vi "Day 5 - If You Give A Seed A Fertilizer.vi"() -> ()   [LabVIEW 2020, in "AoC 2023.lvlib"]
uses:
  AoC 2023.lvlib
  <vilib>/Utility/miscctls.llb/LVMapReplaceAction.ctl
panel:
  out "Puzzle Part-2 Answer":string
  out "Puzzle Answer":string
  in  "Puzzle Input":string="seeds: 79 14 55 13\n\nseed-to-soil map:\n50 98 2\n52 50 48\n\nsoil-to-fertilizer map:\n0 15 37\n37 52 2\n39 0 15\n\nfertilizer-to-water map:\n49 53 8\n0 11 42\n42 0 7\n57 7 4\n\nwater-to-light map:\n88 18 7\n18 25 70\n\nlight-to-temperature map:\n45 77 23\n81 45 19\n68 64 13\n\ntemperature-to-humidity map:\n0 69 1\n1 0 69\n\nhumidity-to-location map:\n60 56 37\n56 93 4"
  # "Enter the Puzzle Input and run the VI"
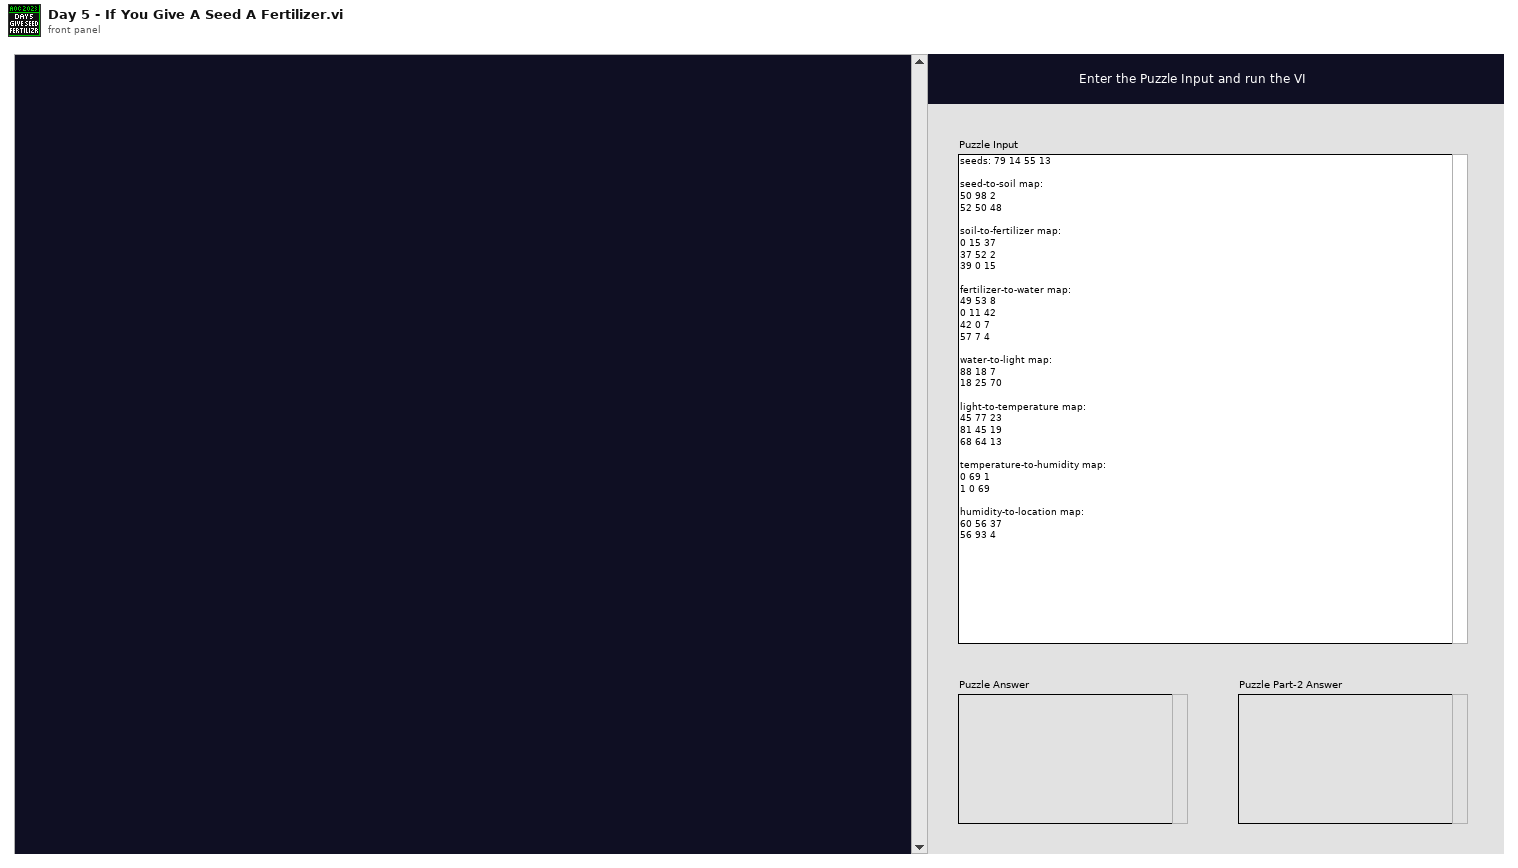
[diagram p1: front panel]
types:
  T1 = map{i32, cluster{"src range start":u64, "src range end":u64, "dst start":u64}[]}
  T2 = typedef "LVMapReplaceAction.ctl" = enum32{"Modify Entry only if found", "Add or Modify Entry", "Delete Entry"}
  T3 = cluster{"src range start":u64, "src range end":u64, "dst start":u64}[]
  T4 = cluster{"src range start":u64, "src range end":u64, "dst start":u64}
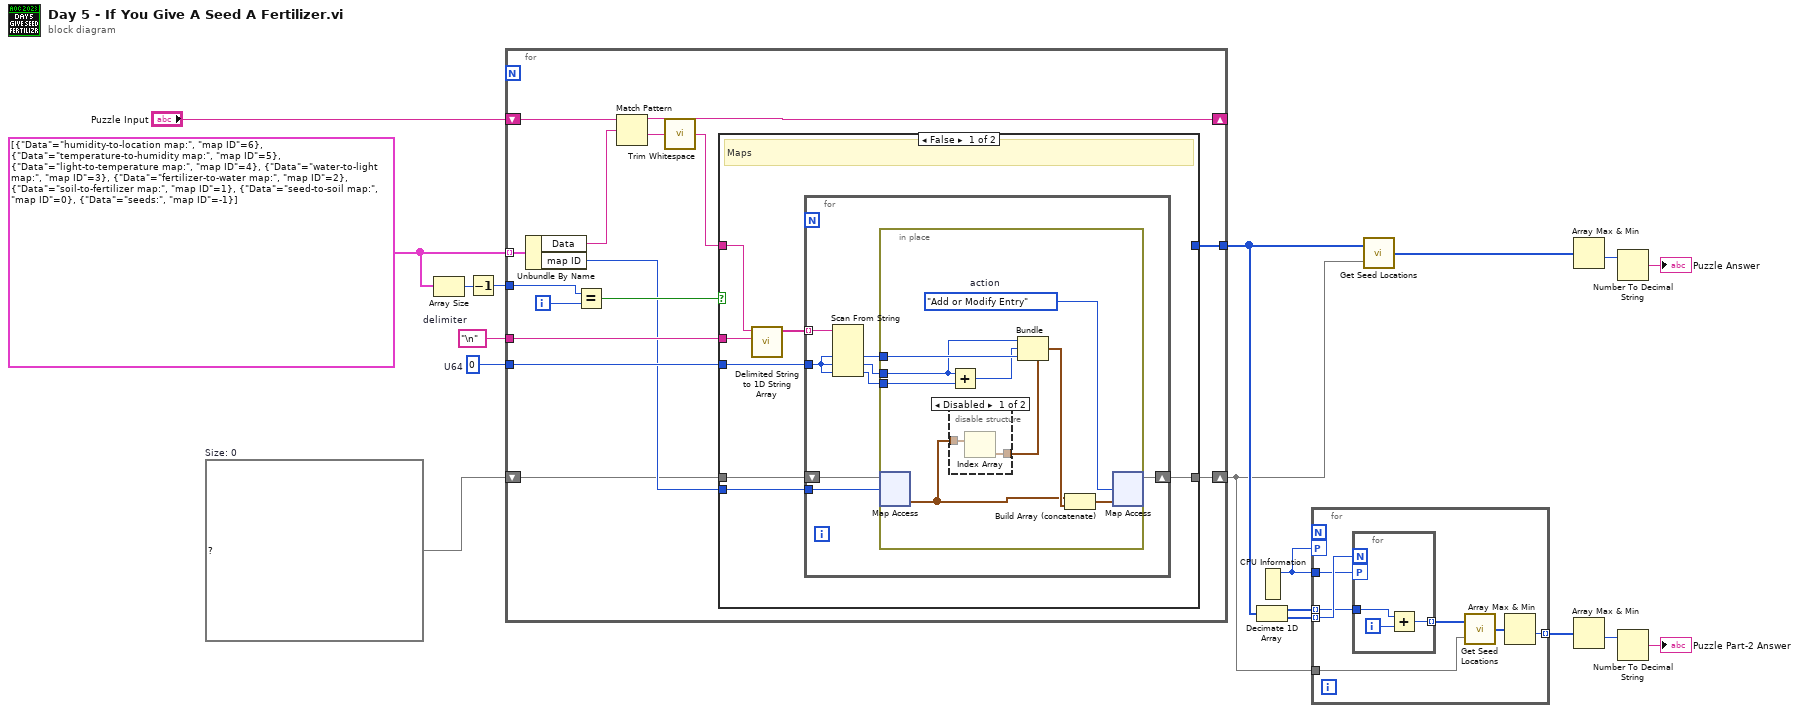
[diagram p0: block diagram]
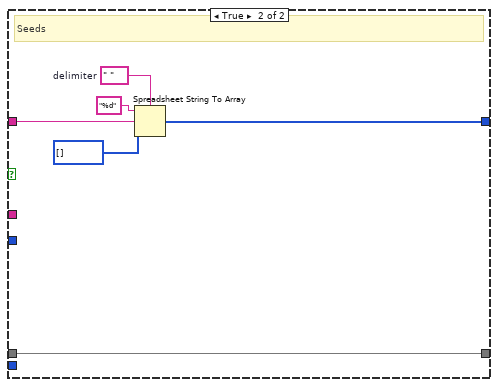
[diagram p3: hidden frame]
diagram:
  w10 = T1 {}  # Size: 0
  w11 = cluster{"Data":string, "map ID":i32}[] [{"Data"="humidity-to-location map:", "map ID"=6}, {"Data"="temperature-to-humidity map:", "map ID"=5}, {"Data"="light-to-temperature map:", "map ID"=4}, {"Data"="water-to-light map:", "map ID"=3}, {"Data"="fertilizer-to-water map:", "map ID"=2}, {"Data"="soil-to-fertilizer map:", "map ID"=1}, {"Data"="seed-to-soil map:", "map ID"=0}, {"Data"="seeds:", "map ID"=-1}]
  w15 = u64 0  # U64
  w16 = "\n"  # delimiter
  n1 = Array Size(array=w11) -> (size(s)=w14:i32)
  n2 = Decrement(x=w14) -> (x-1=w13:i32)
  n3 = for {
    shift-right: [w32] -> _
    shift-left: "Puzzle Input" -> [w33]
    tunnel: w11 -> [w23] mode=indexing
    tunnel: w16 -> [w30]
    tunnel: w15 -> [w28]
    tunnel: w13 -> [w27]
    tunnel: [w24] -> w7
    shift-right: [w20] -> w4
    shift-left: w10 -> [w19]
    i -> [w26]
    n4 = Unbundle By Name(w23) -> ("Data"=w22:string, "map ID"=w21:i32)
    n5 = Equal?(x=w27, y=w26) -> (x = y?=w25:bool)
    n6 = Match Pattern(string=w33, regular expression=w22) -> (before substring=w32:string, after substring=w31:string)  [unwired: 1 in, 2 out]
    n7 = call <vilib>:"Trim Whitespace.vi"("string"=w31) -> ("trimmed string"=w29:string)  [unwired: 1 in]
    n8 = case shown="False" w25 {
      tunnel: w30 -> [w40 _]
      tunnel: w29 -> [w39 w62]
      tunnel: w28 -> [w37 _]
      tunnel: [_ w61] -> w24
      tunnel: w21 -> [w36 _]
      tunnel: [w35 w60] -> w20
      tunnel: w19 -> [w34 w60]
      frame False {
        # "Maps"
        n9 = call <vilib>:"Delimited String to 1D String Array.vi"("delimiter"=w40, "delimited string"=w39) -> ("string array"=w38:string[])  [unwired: 9 in]
        n10 = for {
          tunnel: w38 -> [w48] mode=indexing
          tunnel: w37 -> [w47]
          tunnel: w36 -> [w43]
          shift-right: [w42] -> w35
          shift-left: w34 -> [w41]
          n11 = Scan From String(input string=w48, default 1=w47, default 2=w47, default 3=w47) -> (output 1=w46:u64, output 2=w45:u64, output 3=w44:u64)  [unwired: 3 in, 3 out]
          n12 = in-place {
            in-place-border: w46 -> [w51]
            in-place-border: w45 -> [w50]
            in-place-border: w44 -> [w57]
            w54 = LVMapReplaceAction."Add or Modify Entry"  # action
            n13 = in-place-map #1(w41, w43) -> (w53:T3)  [unwired: 1 in, 1 out]
            n14 = Add(x=w50, y=w57) -> (x+y=w49:u64)
            n15 = disable-structure shown="Disabled" {
              disable-tunnel: w53 -> [w59 _]
              disable-tunnel: [w58 _] -> w52
              frame Disabled {
                n16 = Index Array(array=w59) -> (element=w58:T4)  [unwired: 1 in]
              }
              frame Enabled {
              }
            }
            n17 = Bundle(cluster=w52, "src range start"=w50, "src range end"=w49, "dst start"=w51) -> (w56:T4)
            n18 = Build Array (concatenate)(w53, w56) -> (w55:T3)
            n19 = in-place-map #1(w55, w54) -> (w42:T1)  [unwired: 2 out]
          }
        }
      }
      frame True {
        w65 = " "  # delimiter
        # "Seeds"
        n20 = Spreadsheet String To Array(delimiter (Tab)=w65, format string="%d", spreadsheet string=w62, array type (2D Dbl)=u64[] []) -> (array=w61:u64[])
      }
    }
  }
  n21 = Decimate 1D Array(w7) -> (w6:u64[], w5:u64[])
  n22 = CPU Information() -> (4:w1:i32)  [unwired: 3 out]
  n23 = for {
    tunnel: w6 -> [w71] mode=indexing
    tunnel: w5 -> [w72] mode=indexing
    tunnel: w4 -> [w70]
    tunnel: [w67] -> w3 mode=indexing
    workers-P: w1 -> [_]
    tunnel: w1 -> [w66]
    n24 = for {
      N: w72 -> [_]
      tunnel: w71 -> [w75]
      tunnel: [w73] -> w69 mode=indexing
      workers-P: w66 -> [_]
      i -> [w74]
      n25 = Add(x=w75, y=w74) -> (x+y=w73:u64)
    }
    n26 = call "Get Seed Locations.vi"("Maps"=w70, "Seeds"=w69) -> ("Locations"=w68:u64[])
    n27 = Array Max & Min(array=w68) -> (min value=w67:u64)  [unwired: 3 out]
  }
  n28 = call "Get Seed Locations.vi"("Maps"=w4, "Seeds"=w7) -> ("Locations"=w9:u64[])
  n29 = Array Max & Min(array=w9) -> (min value=w8:u64)  [unwired: 3 out]
  n30 = Array Max & Min(array=w3) -> (min value=w2:u64)  [unwired: 3 out]
  n31 = Number To Decimal String(number=w8) -> (decimal integer string=→"Puzzle Answer":string)  [unwired: 1 in]
  n32 = Number To Decimal String(number=w2) -> (decimal integer string=→"Puzzle Part-2 Answer":string)  [unwired: 1 in]
